vi "T7MOD_Write_UINT16_Registers.vi"(7 "UINT16 to Write":u16[](array[numeric]), 8 "error in":errorcluster, 9 "Starting Address":i32=55110, 10 "Remote Port":u16=502, 11 "Remote IP Address":string="192.168.1.15") -> (0 "error out":errorcluster, 1 "Written At":timestamp)   [LabVIEW 2015]
uses:
  Serial Link Layer/NI_Modbus_Cleaned/NI Modbus121Clean.llb/MB Ethernet Master Query Write Multiple Registers (poly).vi
panel:
  # "Input"
  # "TCP Parameters"
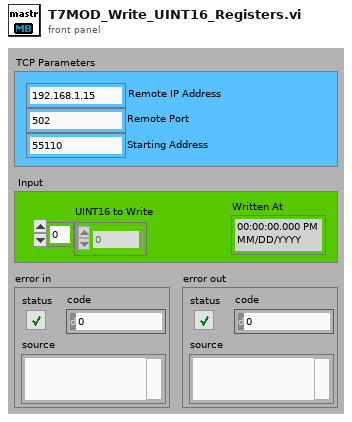
[diagram p1: front panel]
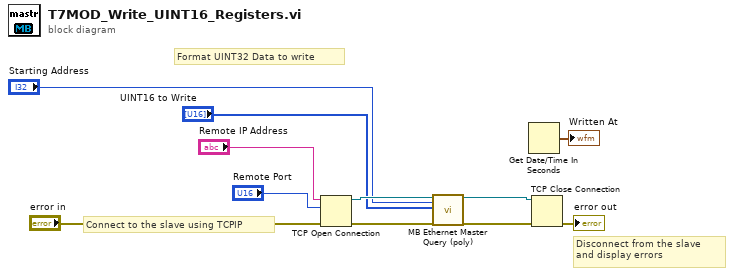
[diagram p0: block diagram]
diagram:
  # "Format UINT32 Data to write"
  # "Disconnect from the slave\nand display errors"
  # "Connect to the slave using TCPIP"
  n1 = TCP Open Connection(address="Remote IP Address", remote port or service name="Remote Port", error in (no error)="error in") -> (connection ID=w9:refnum<k5>, error out=w8:errorcluster)  [unwired: 2 in]
  n2 = call-poly "MB Ethernet Master Query (poly).vi"("TCP Connection Refnum in"=w9, "Starting Address"="Starting Address", "Registers"="UINT16 to Write", "error in"=w8) -> ("TCP Connection Refnum (dup)"=w6:refnum<k5>, "error out"=w7:errorcluster)  [unwired: 13 in, 1 out]
  n3 = Get Date/Time In Seconds() -> (seconds since 1Jan1904=→"Written At":timestamp)
  n4 = TCP Close Connection(connection ID=w6, error in (no error)=w7) -> (error out=→"error out":errorcluster)  [unwired: 2 out]
